vi "Begin.vi"(8 "error in":errorcluster) -> (0 "error out":errorcluster)   [LabVIEW 2016]
doc: "Called before other user functions, this VI is expected to open initial I/O refnums, load in file data, and do all program initialization. Notice that the <B>error out</B> terminal is simply used for data flow. Wiring it to other structures or subVIs ensures that this VI runs first."
uses:
  <vilib>/Rock Robotics/SystemInterfaces/DIO/FPGA_DIOPWMChannel.ctl
  <vilib>/Rock Robotics/WPI/SafetyOutput/WPI_SafetyOutputConfigMenu.ctl
  <vilib>/Rock Robotics/WPI/DriverStation/WPI_DriverStationRobotMode2.ctl
  <vilib>/Rock Robotics/WPI/Joystick/WPI_JoystickDeviceEnum.ctl
  <vilib>/Rock Robotics/SystemInterfaces/DIO/FPGA_DIOChannel.ctl
  <vilib>/Rock Robotics/WPI/Camera/WPI_CameraExposure Values.ctl
  <vilib>/Rock Robotics/WPI/Camera/WPI_CameraFrameRate.ctl
  <vilib>/Rock Robotics/WPI/Camera/WPI_CameraWhite Balance Values.ctl
  <vilib>/Rock Robotics/WPI/Camera/WPI_CameraImageSize.ctl
  <vilib>/Rock Robotics/WPI/RobotDrive/WPI_RobotDriveOpen2MotorWithTalonSRX.vi
  Robot Global Data.vi
  <vilib>/Rock Robotics/Network Tables/NT Write String Array.vi
  <vilib>/Rock Robotics/WPI/MotorControl/WPI_MotorControlOpen TalonSRX.vi
  <vilib>/Rock Robotics/WPI/MotorControl/WPI_MotorControlOpen VictorSP.vi
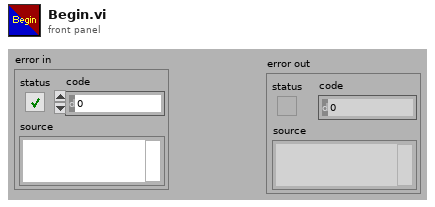
[diagram p1: front panel]
types:
  T1 = typedef "FPGA_DIOPWMChannel.ctl" = enum8{"PWM 0", "PWM 1", "PWM 2", "PWM 3", "PWM 4", "PWM 5", "PWM 6", "PWM 7", "PWM 8", "PWM 9", "PWM MXP 0", "PWM MXP 1", "PWM MXP 2", "PWM MXP 3", "PWM MXP 4", "PWM MXP 5", "PWM MXP 6", "PWM MXP 7", "PWM MXP 8", "PWM MXP 9", "Invalid"}
  T2 = typedef "FPGA_DIOChannel.ctl" = enum8{"DIO 0", "DIO 1", "DIO 2", "DIO 3", "DIO 4", "DIO 5", "DIO 6", "DIO 7", "DIO 8", "DIO 9", "DIO MXP 0", "DIO MXP 1", "DIO MXP 2", "DIO MXP 3", "DIO MXP 4", "DIO MXP 5", "DIO MXP 6", "DIO MXP 7", "DIO MXP 8", "DIO MXP 9", "DIO MXP 10", "DIO MXP 11", "DIO MXP 12", "DIO MXP 13", "DIO MXP 14", "DIO MXP 15", "SPI Port CS1", "SPI Port CS2", "SPI Port CS3", "SPI Port MISO", "SPI Port MOSI", "Invalid"}
  T3 = typedef "WPI_CameraImageSize.ctl" = enum16{"640x480", "320x240", "160x120", "Custom"}
  T4 = typedef "WPI_CameraFrameRate.ctl" = u32
  T5 = typedef "WPI_CameraExposure Values.ctl" = enum16{"Auto", "Flicker-free 50 Hz", "Flicker-free 60 Hz", "Hold current", "Custom"}
  T6 = typedef "WPI_CameraWhite Balance Values.ctl" = enum16{"Auto", "Fixed indoor", "Fixed outdoor 1", "Fixed outdoor 2", "Fixed fluorescent 1", "Fixed fluorescent 2", "Hold current", "Custom"}
  T7 = typedef "WPI_JoystickDeviceEnum.ctl" = enum16{"USB 0", "USB 1", "USB 2", "USB 3", "USB 4", "USB 5"}
  T8 = typedef "WPI_DriverStationRobotMode2.ctl" = enum16{"Autonomous Disabled", "Autonomous Enabled", "Teleop Disabled", "Teleop Enabled", "Disconnected", "Finish", "Test Disabled", "Test Enabled", "Emergency Stopped"}
  T9 = typedef "WPI_SafetyOutputConfigMenu.ctl" = enum16{"Enable", "Disable"}
  T10 = typedef "WPI_JoystickDevRef.ctl" = cluster{"Device":T7}
  T11 = typedef "WPI_RobotDriveDevRef.ctl" = cluster{"DevStatus":errorcluster, "Motors[]":T12[], "Square Inputs":bool, "Max Output":dbl}
  T12 = typedef "WPI_MotorControlDeviceRef.ctl" = cluster{"DeviceStatus":errorcluster, "Type":T13, "PWM":cluster{"PWM Channel":T1, "DeadBand":T14}, "CAN":cluster{"Device Number":u8, "SetOutput VI Ref":variant, "GetOutput VI Ref":variant, "Enable VI Ref":variant, "Disable VI Ref":variant, "Data":variant}, "Invert":bool}
  T13 = typedef "WPI_MotorControlType.ctl" = enum16{"PWM", "CAN"}
  T14 = typedef "WPI_PWMDeadband.ctl" = cluster{"Name":string, "maxPositivePwm":i32, "minPositivePwm":i32, "centerPwm":i32, "maxNegativePwm":i32, "minNegativePwm":i32, "angularRange":u16}
  T15 = typedef "WPI_DigitalInputDevRef.ctl" = cluster{"DevStatus":errorcluster, "DIO Channel":T2}
  T16 = typedef "WPI_CameraDevRef.ctl" = cluster{"Camera Address":string, "CameraStatus":errorcluster}
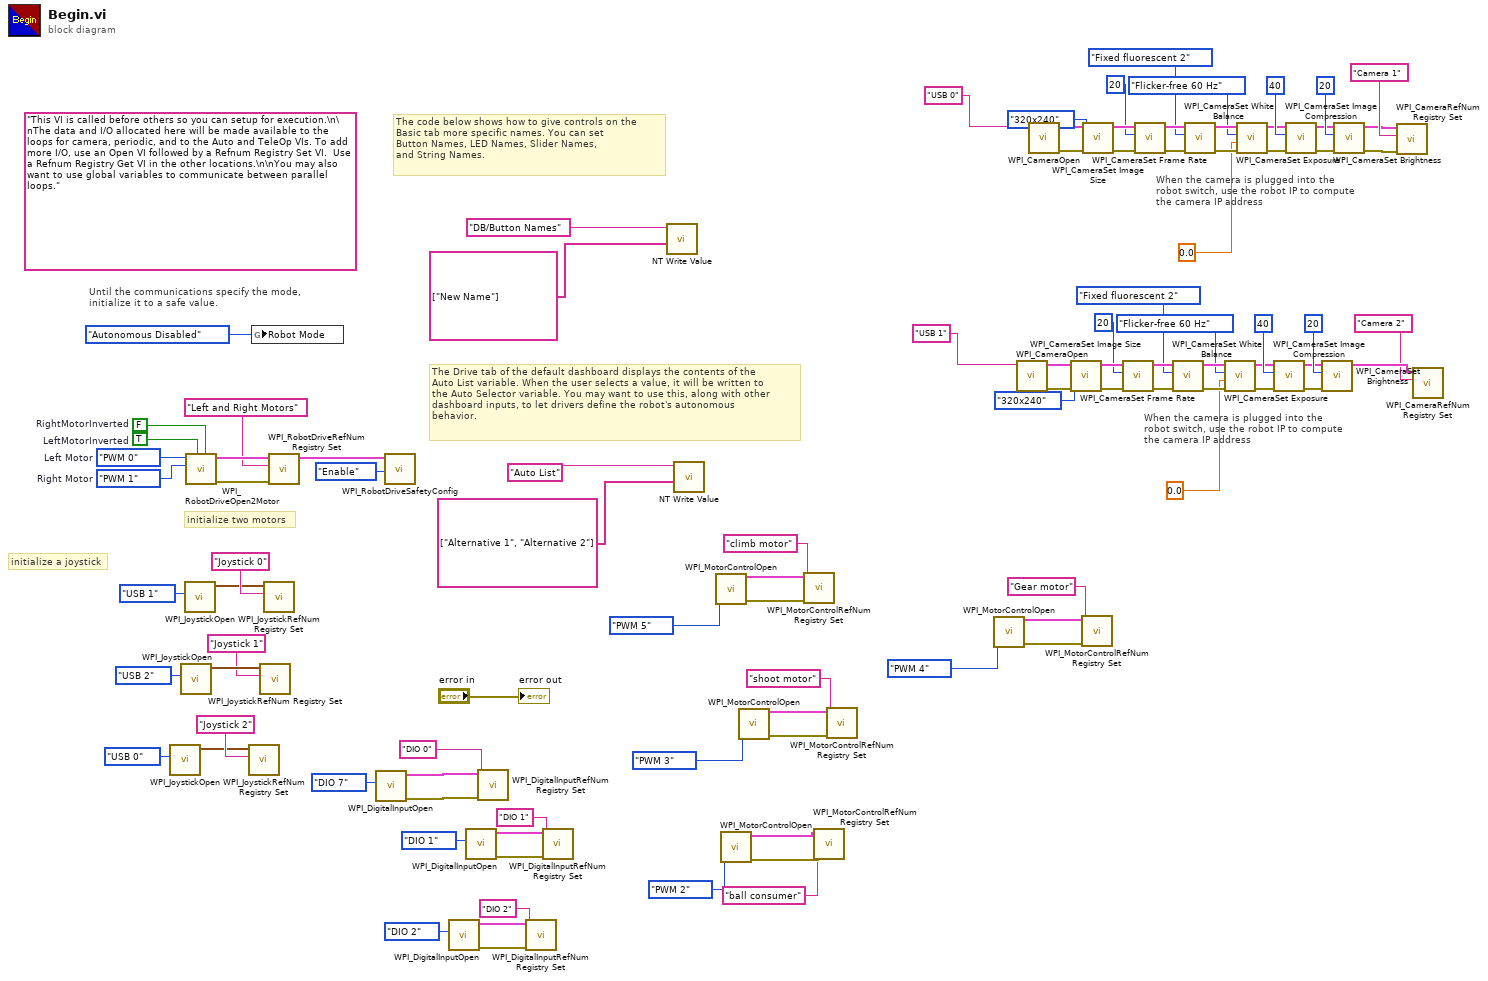
[diagram p0: block diagram]
diagram:
  (unwired) "This VI is called before others so you can setup for execution.\n\nThe data and I/O allocated here will be made available to the loops for camera, periodic, and to the Auto and TeleOp VIs. To add more I/O, use an Open VI followed by a Refnum Registry Set VI.  Use a Refnum Registry Get VI in the other locations.\n\nYou may also want to use global variables to communicate between parallel loops."
  w91 = FPGA_DIOPWMChannel."PWM 1"  # Right Motor
  w92 = FPGA_DIOPWMChannel."PWM 0"  # Left Motor
  w96 = TRUE  # LeftMotorInverted
  w97 = FALSE  # RightMotorInverted
  # "When the camera is plugged into the\nrobot switch, use the robot IP to compute\nthe camera IP address"
  # "When the camera is plugged into the\nrobot switch, use the robot IP to compute\nthe camera IP address"
  # "The Drive tab of the default dashboard displays the contents of the\nAuto List variable. When the user selects a value, it will be written to\nthe Auto Selector variable. You may want to use this, along with other\ndashboard inputs, to let drivers define the robot's autonomous\nbehavior."
  # "The code below shows how to give controls on the\nBasic tab more specific names. You can set\nButton Names, LED Names, Slider Names,\nand String Names."
  # "initialize a joystick"
  # "Until the communications specify the mode,\ninitialize it to a safe value."
  # "initialize two motors"
  n1 = call <vilib>:"WPI_JoystickOpen.vi"("JoystickDevice"=WPI_JoystickDeviceEnum."USB 0") -> ("JoystickDevRef"=w76:T10)  [unwired: 10 in]
  n2 = call <vilib>:"WPI_JoystickOpen.vi"("JoystickDevice"=WPI_JoystickDeviceEnum."USB 2") -> ("JoystickDevRef"=w79:T10)  [unwired: 10 in]
  n3 = call <vilib>:"WPI_JoystickOpen.vi"("JoystickDevice"=WPI_JoystickDeviceEnum."USB 1") -> ("JoystickDevRef"=w86:T10)  [unwired: 10 in]
  n4 = call-poly <vilib>:"WPI_RobotDriveOpen2Motor.vi"("Right Motor Inverted"=w97, "Left Motor Inverted"=w96, "Right Motor"=w91, "Left Motor"=w92) -> ("error out"=w93:errorcluster, "RobotDriveDevRef"=w95:T11)  [unwired: 1 in, 5 out]
  n5 = call <vilib>:"WPI_JoystickRefNum Registry Set.vi"("refnum name"="Joystick 2", "JoystickDevRef"=w76) -> ()  [unwired: 8 in, 2 out]
  n6 = global write "Robot Global Data.vi" "Robot Mode"(WPI_DriverStationRobotMode2."Autonomous Disabled" ("Robot Mode")) -> ()
  n7 = call <vilib>:"WPI_JoystickRefNum Registry Set.vi"("refnum name"="Joystick 1", "JoystickDevRef"=w79) -> ()  [unwired: 8 in, 2 out]
  n8 = call <vilib>:"WPI_JoystickRefNum Registry Set.vi"("refnum name"="Joystick 0", "JoystickDevRef"=w86) -> ()  [unwired: 8 in, 2 out]
  n9 = call <vilib>:"WPI_RobotDriveRefNum Registry Set.vi"("error in (no error)"=w93, "refnum name"="Left and Right Motors", "RobotDriveDevRef"=w95) -> ("RobotDriveDevRef"=w90:T11)  [unwired: 1 in, 7 out]
  n10 = call <vilib>:"WPI_DigitalInputOpen.vi"("DIO Channel"=FPGA_DIOChannel."DIO 7") -> ("error out"=w61:errorcluster, "DigitalInputDevRef"=w62:T15)  [unwired: 9 in]
  n11 = call <vilib>:"WPI_RobotDriveSafetyConfig.vi"("mode"=WPI_SafetyOutputConfigMenu."Enable", "RobotDriveDevRef"=w90) -> ()  [unwired: 8 in, 2 out]
  n12 = call <vilib>:"WPI_DigitalInputOpen.vi"("DIO Channel"=FPGA_DIOChannel."DIO 2") -> ("error out"=w7:errorcluster, "DigitalInputDevRef"=w6:T15)  [unwired: 9 in]
  n13 = call <vilib>:"WPI_DigitalInputOpen.vi"("DIO Channel"=FPGA_DIOChannel."DIO 1") -> ("error out"=w58:errorcluster, "DigitalInputDevRef"=w57:T15)  [unwired: 9 in]
  n14 = call <vilib>:"WPI_DigitalInputRefNum Registry Set.vi"("error in (no error)"=w61, "refnum name"="DIO 0", "DigitalInputDevRef"=w62) -> ()  [unwired: 7 in, 2 out]
  n15 = call <vilib>:"WPI_DigitalInputRefNum Registry Set.vi"("error in (no error)"=w7, "refnum name"="DIO 2", "DigitalInputDevRef"=w6) -> ()  [unwired: 7 in, 2 out]
  n16 = call <vilib>:"WPI_DigitalInputRefNum Registry Set.vi"("error in (no error)"=w58, "refnum name"="DIO 1", "DigitalInputDevRef"=w57) -> ()  [unwired: 7 in, 2 out]
  n17 = call-poly <vilib>:"NT Write Value.vi"("String Array"=string[] ["New Name"], "Name"="DB/Button Names") -> ()  [unwired: 9 in, 1 out]
  n18 = call-poly <vilib>:"NT Write Value.vi"("String Array"=string[] ["Alternative 1", "Alternative 2"], "Name"="Auto List") -> ()  [unwired: 9 in, 1 out]
  n19 = call-poly <vilib>:"WPI_MotorControlOpen.vi"("PWM Channel"=FPGA_DIOPWMChannel."PWM 5") -> ("error out"=w73:errorcluster, "MotorControlDeviceRef"=w72:T12)  [unwired: 9 in]
  n20 = call-poly <vilib>:"WPI_MotorControlOpen.vi"("PWM Channel"=FPGA_DIOPWMChannel."PWM 2") -> ("error out"=w3:errorcluster, "MotorControlDeviceRef"=w4:T12)  [unwired: 9 in]
  n21 = call-poly <vilib>:"WPI_MotorControlOpen.vi"("PWM Channel"=FPGA_DIOPWMChannel."PWM 3") -> ("error out"=w68:errorcluster, "MotorControlDeviceRef"=w69:T12)  [unwired: 9 in]
  n22 = call <vilib>:"WPI_MotorControlRefNum Registry Set.vi"("error in (no error)"=w73, "refnum name"="climb motor", "MotorControlDevRef"=w72) -> ()  [unwired: 7 in, 2 out]
  n23 = call <vilib>:"WPI_MotorControlRefNum Registry Set.vi"("error in (no error)"=w3, "refnum name"="ball consumer", "MotorControlDevRef"=w4) -> ()  [unwired: 7 in, 2 out]
  n24 = call <vilib>:"WPI_MotorControlRefNum Registry Set.vi"("error in (no error)"=w68, "refnum name"="shoot motor", "MotorControlDevRef"=w69) -> ()  [unwired: 7 in, 2 out]
  n25 = call-poly <vilib>:"WPI_MotorControlOpen.vi"("PWM Channel"=FPGA_DIOPWMChannel."PWM 4") -> ("error out"=w65:errorcluster, "MotorControlDeviceRef"=w64:T12)  [unwired: 9 in]
  n26 = call <vilib>:"WPI_CameraOpen.vi"("Camera Address"="USB 1" ("format string")) -> ("error out"=w24:errorcluster, "CameraDevRef"=w25:T16)  [unwired: 1 in, 8 out]
  n27 = call <vilib>:"WPI_CameraOpen.vi"("Camera Address"="USB 0" ("format string")) -> ("error out"=w44:errorcluster, "CameraDevRef"=w45:T16)  [unwired: 1 in, 8 out]
  n28 = call <vilib>:"WPI_CameraSet Image Size.vi"("error in (no error)"=w24, "Image Size"=WPI_CameraImageSize."320x240", "CameraDevRef"=w25) -> ("error out"=w23:errorcluster, "CameraDevRef Out"=w26:T16)  [unwired: 1 in, 6 out]
  n29 = call <vilib>:"WPI_MotorControlRefNum Registry Set.vi"("error in (no error)"=w65, "refnum name"="Gear motor", "MotorControlDevRef"=w64) -> ()  [unwired: 7 in, 2 out]
  n30 = call <vilib>:"WPI_CameraSet Image Size.vi"("error in (no error)"=w44, "Image Size"=WPI_CameraImageSize."320x240", "CameraDevRef"=w45) -> ("error out"=w43:errorcluster, "CameraDevRef Out"=w46:T16)  [unwired: 1 in, 6 out]
  n31 = call <vilib>:"WPI_CameraSet Frame Rate.vi"("error in (no error)"=w23, "Frame Rate (fps)"=T4 20, "CameraDevRef"=w26) -> ("error out"=w22:errorcluster, "CameraDevRef Out"=w28:T16)  [unwired: 7 out]
  n32 = call <vilib>:"WPI_CameraSet Frame Rate.vi"("error in (no error)"=w43, "Frame Rate (fps)"=T4 20, "CameraDevRef"=w46) -> ("error out"=w42:errorcluster, "CameraDevRef Out"=w48:T16)  [unwired: 7 out]
  n33 = call <vilib>:"WPI_CameraSet White Balance.vi"("error in (no error)"=w22, "White Balance"=WPI_CameraWhite_Balance_Values."Fixed fluorescent 2", "CameraDevRef"=w28) -> ("error out"=w21:errorcluster, "CameraDevRef Out"=w27:T16)  [unwired: 1 in, 6 out]
  n34 = call <vilib>:"WPI_CameraSet White Balance.vi"("error in (no error)"=w42, "White Balance"=WPI_CameraWhite_Balance_Values."Fixed fluorescent 2", "CameraDevRef"=w48) -> ("error out"=w41:errorcluster, "CameraDevRef Out"=w47:T16)  [unwired: 1 in, 6 out]
  n35 = call <vilib>:"WPI_CameraSet Exposure.vi"("error in (no error)"=w21, "Exposure (%)"=0.0, "Exposure"=WPI_CameraExposure_Values."Flicker-free 60 Hz", "CameraDevRef"=w27) -> ("error out"=w20:errorcluster, "CameraDevRef Out"=w30:T16)  [unwired: 6 out]
  n36 = call <vilib>:"WPI_CameraSet Exposure.vi"("error in (no error)"=w41, "Exposure (%)"=0.0, "Exposure"=WPI_CameraExposure_Values."Flicker-free 60 Hz", "CameraDevRef"=w47) -> ("error out"=w40:errorcluster, "CameraDevRef Out"=w50:T16)  [unwired: 6 out]
  n37 = call <vilib>:"WPI_CameraSet Image Compression.vi"("error in (no error)"=w20, "Compression"=40, "CameraDevRef"=w30) -> ("error out"=w19:errorcluster, "CameraDevRef Out"=w29:T16)  [unwired: 7 out]
  n38 = call <vilib>:"WPI_CameraSet Image Compression.vi"("error in (no error)"=w40, "Compression"=40, "CameraDevRef"=w50) -> ("error out"=w39:errorcluster, "CameraDevRef Out"=w49:T16)  [unwired: 7 out]
  n39 = call <vilib>:"WPI_CameraSet Brightness.vi"("error in (no error)"=w19, "Brightness"=20, "CameraDevRef"=w29) -> ("CameraDevRef Out"=w12:T16)  [unwired: 8 out]
  n40 = call <vilib>:"WPI_CameraSet Brightness.vi"("error in (no error)"=w39, "Brightness"=20, "CameraDevRef"=w49) -> ("error out"=w33:errorcluster, "CameraDevRef Out"=w34:T16)  [unwired: 7 out]
  n41 = call <vilib>:"WPI_CameraRefNum Registry Set.vi"("error in (no error)"=w33, "refnum name"="Camera 1", "CameraDevRef"=w34) -> ()  [unwired: 1 in, 8 out]
  n42 = call <vilib>:"WPI_CameraRefNum Registry Set.vi"("refnum name"="Camera 2", "CameraDevRef"=w12) -> ()  [unwired: 2 in, 8 out]
  "error out" <- "error in"
